vi "D2SParser - Private - Helper - Read Bits.vi"(8 "error in (no error)":errorcluster, 9 "# Bits":i32, 10 "Position":i64, 11 "D2SParser in":refnum<class "D2SParser.lvclass">) -> (0 "error out":errorcluster, 2 "bits":bool[](array[boolean]), 3 "D2SParser out":refnum<class "D2SParser.lvclass">)   [LabVIEW 2015, in "D2SParser.lvclass"]
uses:
  D2SParser.lvclass
  D2SParser.lvclass/D2SParser.ctl
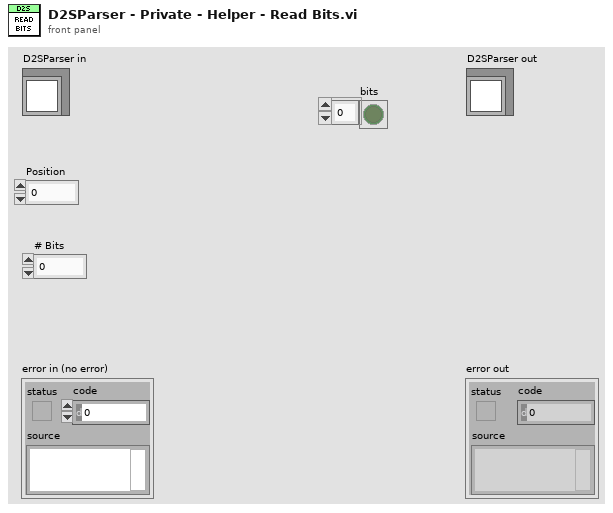
[diagram p1: front panel]
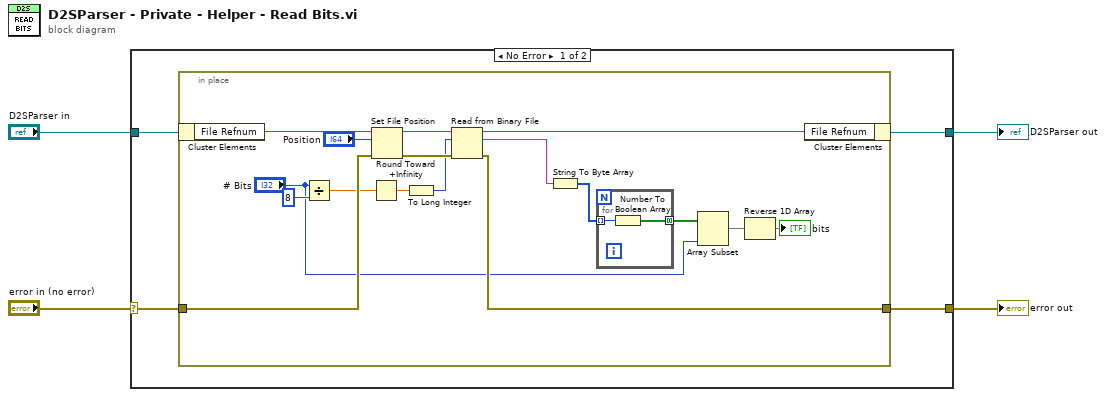
[diagram p0: block diagram]
diagram:
  n1 = case shown="No Error" "error in (no error)" {
    selector: "error in (no error)" -> [w7 w29]
    tunnel: [w6 w29] -> w3
    tunnel: [w5 w28] -> w1
    tunnel: "D2SParser in" -> [w8 w28]
    frame No Error {
      n2 = in-place {
        in-place-border: w7 -> [w21]
        in-place-border: [w19] -> w6
        n3 = in-place-cluster #1(w8) -> ("File Refnum"=w23:refnum<file>)
        n4 = Divide(x="# Bits", y=8) -> (x/y=w18:dbl)
        n5 = Round Toward +Infinity(x=w18) -> (ceil(x): smallest int >= x=w16:dbl)
        n6 = Set File Position(offset (in bytes) (0)="Position", refnum=w23, error in=w21) -> (refnum out=w24:refnum<file>, error out=w25:errorcluster)  [unwired: 1 in]
        n7 = To Long Integer(number=w16) -> (32bit integer=w15:i32)
        n8 = Read from Binary File(8:w25, 10:w15, 11:w24) -> (0:w19:errorcluster, 2:w14:string, 3:w22:refnum<file>)  [unwired: 3 in, 1 out]
        n9 = String To Byte Array(string=w14) -> (unsigned byte array=w13:u8[])
        n10 = for {
          tunnel: w13 -> [w27] mode=indexing
          tunnel: [w26] -> w12 mode=concatenating
          n11 = Number To Boolean Array(number=w27) -> (Boolean array=w26:bool[])
        }
        n12 = Array Subset(array=w12, length="# Bits") -> (w10:bool[])  [unwired: 1 in]
        n13 = Reverse 1D Array(array=w10) -> (reversed array=→"bits":bool[])
        n14 = in-place-cluster #1("File Refnum"=w22) -> (w5:refnum<class "D2SParser.lvclass">)
      }
    }
    frame Error {
    }
  }
  "error out" <- w3
  "D2SParser out" <- w1
